vi "全局 3.vi"() -> ()   [LabVIEW 2013]
panel:
  out "产品":string
  in  "步骤 3":bool[](array[boolean])
  in  "步骤 2":bool[](array[boolean])
  in  "VIRef引用句柄":refnum<vi>
  in  "步骤":bool[](array[boolean])
  in  "总合格状态":string
  in  "合格判断":string
  in  "stop":bool
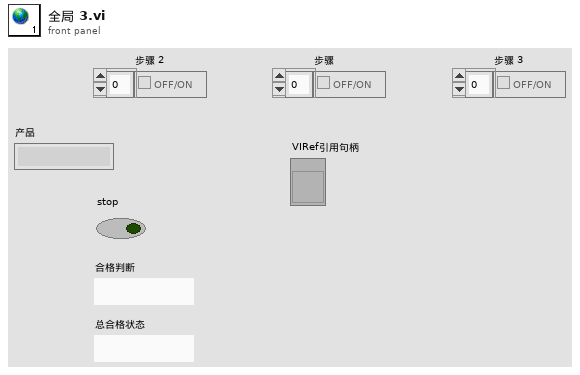
[diagram p1: front panel]
diagram:
